vi "RotateArrayInRadians.vi"(8 "X, Y, Z Input":dbl[](array[numeric]) format="%#_13g", 11 "Angle":dbl) -> (0 "X', Y', Z Output":dbl[](array[numeric]))   [LabVIEW 2016]
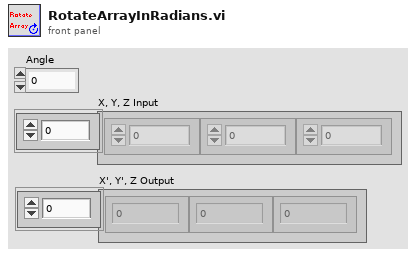
[diagram p1: front panel]
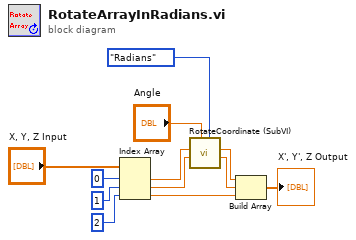
[diagram p0: block diagram]
diagram:
  n1 = Index Array(array="X, Y, Z Input", index #1=0 ("index"), index #2=1 ("index"), index #3=2 ("index")) -> (element #1=w9:dbl, element #2=w10:dbl, element #3=w1:dbl)
  n2 = call "RotateCoordinate (SubVI).vi"("Units"=enum16{"mrad", "Radians", "Degrees"}."Radians", "Angle"="Angle", "y"=w10, "x"=w9) -> ("y'"=w4:dbl, "x'"=w5:dbl)  [unwired: 5 in, 1 out]
  n3 = Build Array(w5, w4, w1) -> (→"X', Y', Z Output":dbl[])
